vi "CompVisionUtil_EstimateFieldToCamera.vi"(9 "FieldToTarget":T1={"TRANSLATION"={"X"=0.0, "Y"=0.0}, "ROTATION"={"VALUE"=0.0, "COS"=1.0, "SIN"=0.0}} {"ROTATION"."SIN" format="%13.4f"; "ROTATION"."COS" format="%13.4f"; "ROTATION"."VALUE" format="%13.4f"; "TRANSLATION"."Y" format="%14.3f"; "TRANSLATION"."X" format="%14.3f"}, 11 "CameraToTarget":T4={"TRANSLATION"={"X"=0.0, "Y"=0.0}, "ROTATION"={"VALUE"=0.0, "COS"=1.0, "SIN"=0.0}, "xF"=FALSE} {"ROTATION"."SIN" format="%13.4f"; "ROTATION"."COS" format="%13.4f"; "ROTATION"."VALUE" format="%13.4f"; "TRANSLATION"."Y" format="%14.3f"; "TRANSLATION"."X" format="%14.3f"}) -> (3 "EstimateFieldToCamera":T1={"TRANSLATION"={"X"=0.0, "Y"=0.0}, "ROTATION"={"VALUE"=0.0, "COS"=1.0, "SIN"=0.0}} {"ROTATION"."SIN" format="%13.4f"; "ROTATION"."COS" format="%13.4f"; "ROTATION"."VALUE" format="%13.4f"; "TRANSLATION"."Y" format="%14.3f"; "TRANSLATION"."X" format="%14.3f"})   [LabVIEW 2019, in "Trajectory_Library.lvlib"]
doc: "Estimates the pose of the camera in the field coordinate system, given the position of the target relative to the camera, and the target relative to the field. This *only* tracks the position of the camera, not the position of the robot itself.\n\nInputs:\n -- CameraToTarget -- Transform containing the position of the target relative to the camera.\n -- FieldToTarget -- Pose containing the position of the target in the field.\n\nOutput:\n -- EstimateFieldToCamera -- Pose containing position of the camera in the field."
uses:
  Trajectory_Library.lvlib
  TypeDef/TRANSFORM2D.ctl
  TypeDef/TRANSLATION2D.ctl
  TypeDef/ROTATION2D.ctl
  TypeDef/POSE2D.ctl
  Transform2d_Create_TransRot.vi
  Translation2d_UnaryMinus.vi
  Rotation2d_UnaryMinus.vi
  Translation2d_RotateBy.vi
  Translation2d_Plus.vi
  Rotation2d_Plus.vi
  Pose2d_New_TRRO.vi
  Translation2d_Create.vi
  Rotation2d_CreateAngle.vi
  Rotation2d_RotateBy.vi
  Rotation2d_CreateXY.vi
  Util_CalcDist.vi
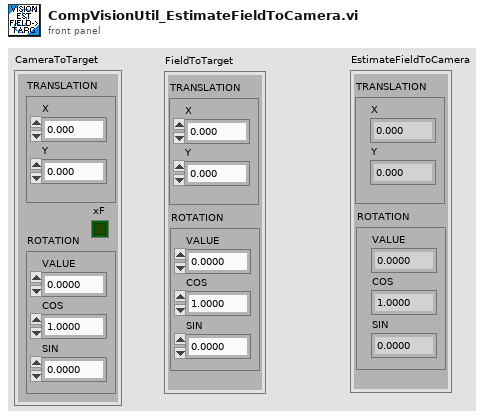
[diagram p1: front panel]
types:
  T1 = typedef "Trajectory_Library.lvlib/POSE2D.ctl" = cluster{"TRANSLATION":T2, "ROTATION":T3}
  T2 = typedef "Trajectory_Library.lvlib/TRANSLATION2D.ctl" = cluster{"X":dbl, "Y":dbl}
  T3 = typedef "Trajectory_Library.lvlib/ROTATION2D.ctl" = cluster{"VALUE":dbl, "COS":dbl, "SIN":dbl}
  T4 = typedef "Trajectory_Library.lvlib/TRANSFORM2D.ctl" = cluster{"TRANSLATION":T2, "ROTATION":T3, "xF":bool}
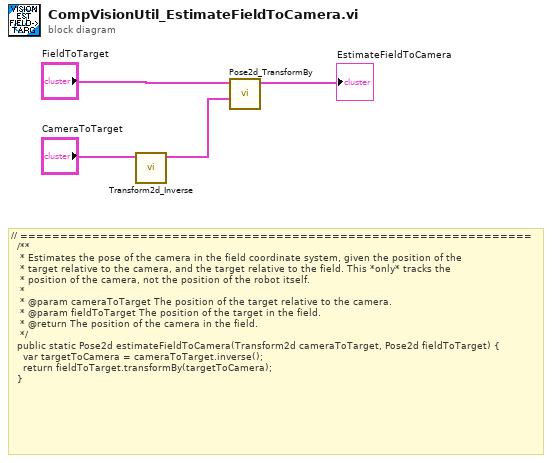
[diagram p0: block diagram]
diagram:
  # "// ================================================================\n  /**\n   * Estimates the pose of the camera in the field coordinate system, given the position of the\n   * target relative to the camera, and the target relative to the field. This *only* tracks the\n   * position of the camera, not the position of the robot itself.\n   *\n   * @param cameraToTarget The position of the target relative to the camera.\n   * @param fieldToTarget The position of the target in the field.\n   * @return The position of the camera in the field.\n   */\n  public static Pose2d estimateFieldToCamera(Transform2d cameraToTarget, Pose2d fieldToTarget) {\n    var targetToCamera = cameraToTarget.inverse();\n    return fieldToTarget.transformBy(targetToCamera);\n  }"
  n1 = call "Transform2d_Inverse.vi"("inTRANSFORM"="CameraToTarget") -> ("TRANSFORM"=w2:T4)  [unwired: 10 in]
  n2 = call "Pose2d_TransformBy.vi"("other TRANSFORM"=w2, "in POSE"="FieldToTarget") -> ("out POSE"=→"EstimateFieldToCamera":T1)  [unwired: 9 in]
